vi "Configure Basic Analog Generator.vi"(0 "VISA resource name":refnum<visa-resource-name>, 1 "Sample Rate (0: agHz512k)":i32(ring) items=["agHz512k", "agHz128k", "agHz64k", "agOSR", "agISR"], 2 "Auto On (T: Enable)":bool=TRUE, 5 "Connector Configuration (0: aoUnbalGnd)":i32(ring) items=["aoUnbalGnd", "aoUnbalFloat", "aoBalGnd", "aoBalFloat", "aoBalCommon"], 7 "Output Impedance (0: aozBal50Un25)":i32(ring) items=["aozBal50Un25", "aozBal150Un75", "aoz600"], 9 "Output Mode (0: Stereo)":i32(ring) items=["Stereo", "Mono"], 11 "error in (no error)":errorcluster, 12 "AB Lock (T: Enable)":bool=TRUE, 13 "Invert EQ (T: Enable)":bool=TRUE) -> (4 "VISA resource name out":refnum<visa-resource-name>, 15 "error out":errorcluster)   [LabVIEW 2014, in "Stanford Research SR1.lvlib"]
doc: "Configures the basic attributes for the Analog Generator."
uses:
  Stanford Research SR1.lvlib
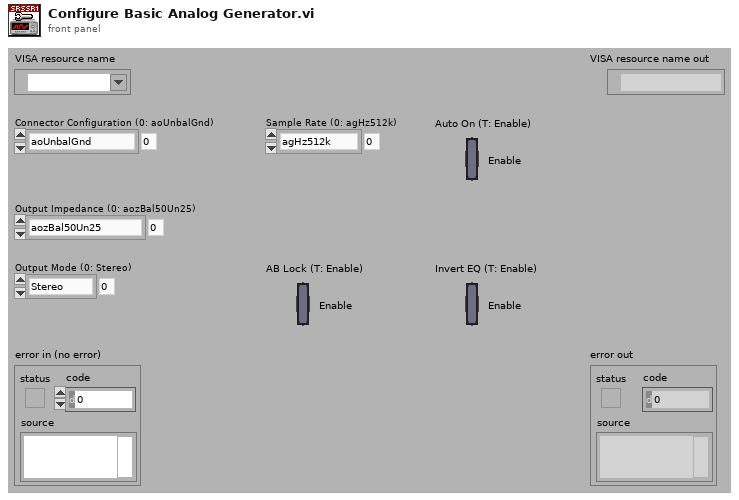
[diagram p1: front panel]
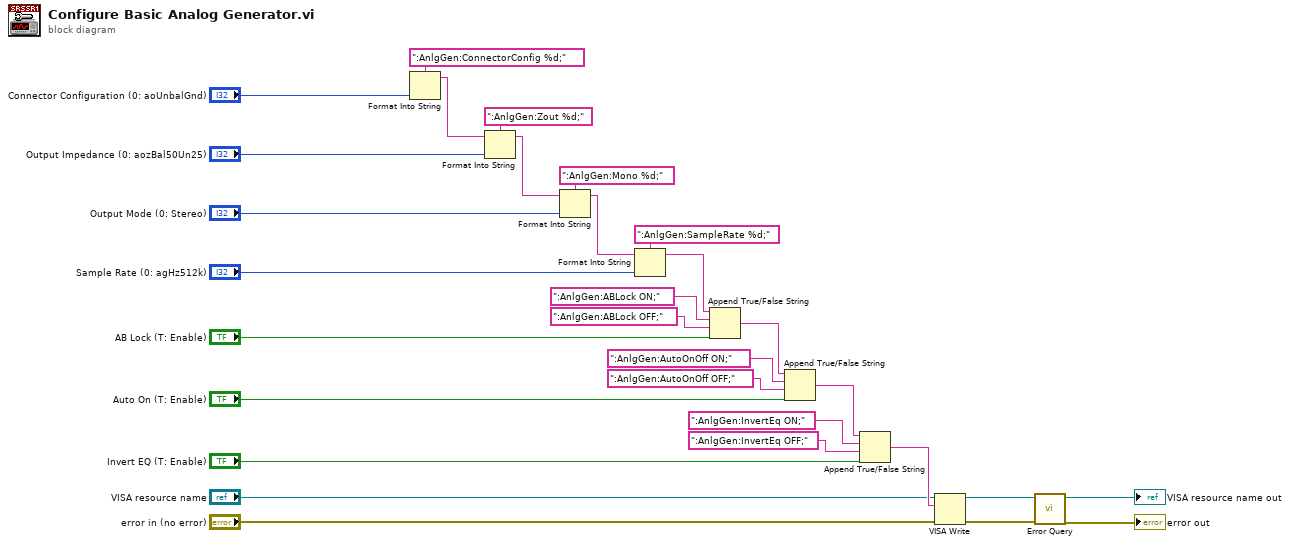
[diagram p0: block diagram]
diagram:
  n1 = Format Into String(format string=":AnlgGen:ConnectorConfig %d;", "Connector Configuration (0: aoUnbalGnd)") -> (resulting string=w28:string)  [unwired: 2 in, 1 out]
  n2 = Format Into String(format string=":AnlgGen:Zout %d;", initial string=w28, "Output Impedance (0: aozBal50Un25)") -> (resulting string=w25:string)  [unwired: 1 in, 1 out]
  n3 = Format Into String(format string=":AnlgGen:Mono %d;", initial string=w25, "Output Mode (0: Stereo)") -> (resulting string=w22:string)  [unwired: 1 in, 1 out]
  n4 = Format Into String(format string=":AnlgGen:SampleRate %d;", initial string=w22, "Sample Rate (0: agHz512k)") -> (resulting string=w19:string)  [unwired: 1 in, 1 out]
  n5 = Append True/False String(1:"AB Lock (T: Enable)", 2:":AnlgGen:ABLock OFF;", 3:":AnlgGen:ABLock ON;", 4:w19) -> (0:w15:string)
  n6 = Append True/False String(1:"Auto On (T: Enable)", 2:":AnlgGen:AutoOnOff OFF;", 3:":AnlgGen:AutoOnOff ON;", 4:w15) -> (0:w11:string)
  n7 = Append True/False String(1:"Invert EQ (T: Enable)", 2:":AnlgGen:InvertEq OFF;", 3:":AnlgGen:InvertEq ON;", 4:w11) -> (0:w7:string)
  n8 = VISA Write(VISA resource name="VISA resource name", write buffer=w7, error in (no error)="error in (no error)") -> (VISA resource name out=w4:refnum<visa-resource-name>, error out=w3:errorcluster)  [unwired: 1 out]
  n9 = call "Error Query.vi"("error in (no error)"=w3, "VISA resource name"=w4) -> ("error out"=→"error out":errorcluster, "VISA resource name out"=→"VISA resource name out":refnum<visa-resource-name>)  [unwired: 6 in, 2 out]
